vi "Lockin.Read Configuration.vi"(8 "error in (no error)":errorcluster, 11 "Instrument.Lockin":refnum<class "Instrument.Lockin.lvclass">) -> (0 "error out":errorcluster, 2 "Configuration":T1={"Channels: AO"={"Ch"=[], "Amp (V)"=[], "DC (V)"=[], "f (Hz)"=[], "Phase (°)"=[], "Function"=[], "Sweep?"=[]}, "Channels: REF"={"Ch"=[13], " f (Hz)"=[], "Phase (°)"=[], "TC (s)"=[0.0], "order"=[0]}, "REF Filter"={"60 Hz prefilter"=FALSE, "LP prefilter"=FALSE, "LP cutoff (Hz)"=0.0}, "Amplifers"={"offsets"=[], "Gain"=[], "Amplifiers"=enum."Manual"}, "DAQ"={"sampling"={"Fs"=0.0, "#s"=500}, "sample mode"=10178, "buffer size (S)"=0, "decimation"=0}, "Calibration"={"Cal Info"=[]}, "AI Configuration"=[], "AO Configuration"=[], "Aux Channel"="Dev2/ao0"} {"AO Configuration"."output terminal configuration" items=["Default"=-1, "RSE"=10083, "Differential"=10106, "Pseudodifferential"=12529]; "AI Configuration"."input terminal configuration" items=["default"=-1, "RSE"=10083, "NRSE"=10078, "Differential"=10106, "Pseudodifferential"=12529]; "AI Configuration"."AI.Coupling" items=["AC"=10045, "DC"=10050, "GND"=10066]; "DAQ"."sample mode" items=["Finite Samples"=10178, "Continuous Samples"=10123]; "Channels: AO"."f (Hz)" min=0.001 max=10000.0 format="%.3g"; "Channels: AO"."Phase (°)" format="%.3g"; "Channels: AO"."DC (V)" format="%.3p"; "Channels: AO"."Amp (V)" min=0.0 max=10.0 format="%.3p"; "Channels: REF"."order" min=1; "Channels: REF"."TC (s)" min=1e-05 format="%#_3p"; "Channels: REF"."Phase (°)" format="%.3g"; "Channels: REF"."f (Hz)" format="%.3g"}, 3 "Instrument.Lockin out":refnum<class "Instrument.Lockin.lvclass">)   [LabVIEW 2016, in "Instrument.Lockin.lvclass"]
uses:
  Instrument.Lockin.lvclass
  Typedefs/Lockin.Configuration--Cluster.ctl
  LockinDAQ/Typedefs/AO-cluster.ctl
  LockinDAQ/Typedefs/Function-enum.ctl
  LockinDAQ/Typedefs/REF-cluster.ctl
  LockinDAQ/Typedefs/AI Prefilter-cluster.ctl
  LockinDAQ/Typedefs/AmplifierType-enum.ctl
  LockinDAQ/Typedefs/Sampling.ctl
  LockinDAQ/Typedefs/Cal Info - Cluster.ctl
  LockinDAQ/Typedefs/AI.config-array.ctl
  LockinDAQ/Typedefs/AI.config-cluster.ctl
  LockinDAQ/Typedefs/AI.coupling-enum.ctl
  LockinDAQ/Typedefs/446xAI-enum.ctl
  LockinDAQ/Typedefs/DAQType-enum.ctl
  LockinDAQ/Typedefs/AO.config-array.ctl
  LockinDAQ/Typedefs/AO.config-cluster.ctl
  LockinDAQ/Typedefs/446xAO-enum.ctl
  Instrument.Lockin.lvclass/Instrument.Lockin.ctl
  LockinDAQ/LockinDAQ.lvclass
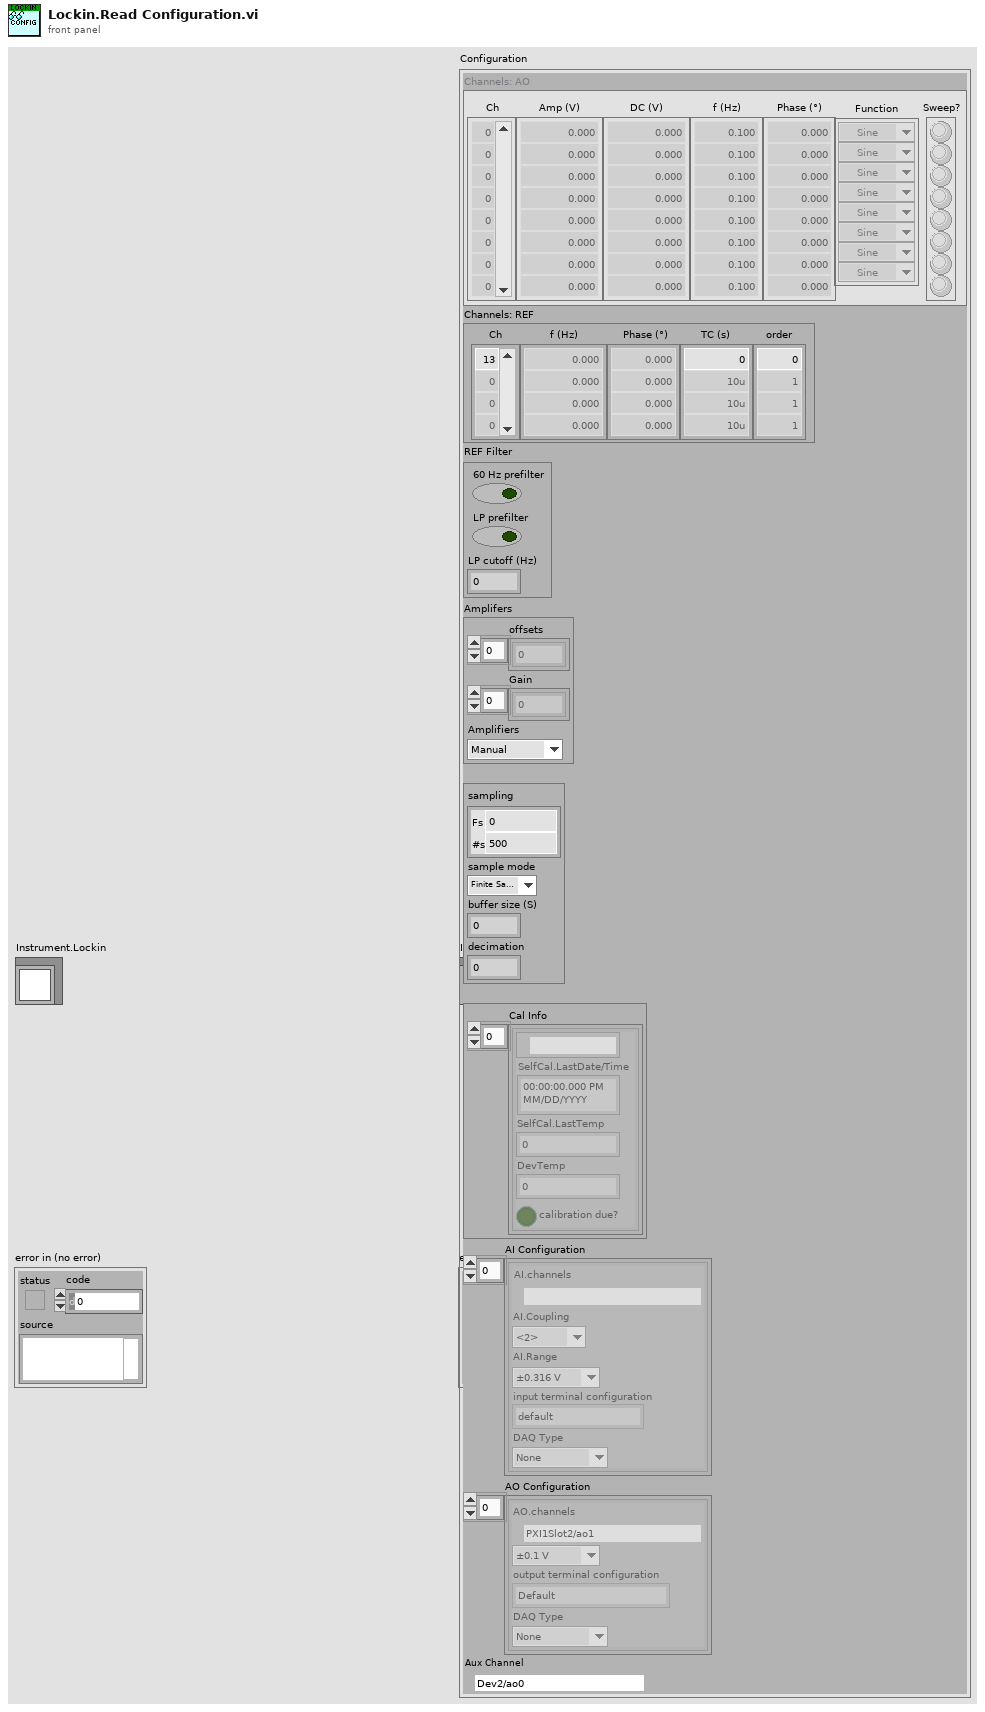
[diagram p1: front panel]
types:
  T1 = typedef "Instrument.Lockin.lvclass/Lockin.Configuration--Cluster.ctl" = cluster{"Channels: AO":T2, "Channels: REF":T4, "REF Filter":T5, "Amplifers":cluster{"offsets":dbl[], "Gain":dbl[], "Amplifiers":T6}, "DAQ":cluster{"sampling":T7, "sample mode":i32, "buffer size (S)":u32, "decimation":u32}, "Calibration":cluster{"Cal Info":T8[]}, "AI Configuration":T9, "AO Configuration":T14, "Aux Channel":tag}
  T2 = typedef "LockinDAQ.lvclass/AO-cluster.ctl" = cluster{"Ch":i32[], "Amp (V)":dbl[], "DC (V)":dbl[], "f (Hz)":dbl[], "Phase (°)":dbl[], "Function":T3[], "Sweep?":bool[]}
  T3 = typedef "LockinDAQ.lvclass/Function-enum.ctl" = enum16{"Sine", "Triangle", "Square", "Sawtooth"}
  T4 = typedef "LockinDAQ.lvclass/REF-cluster.ctl" = cluster{"Ch":i32[], " f (Hz)":dbl[], "Phase (°)":dbl[], "TC (s)":dbl[], "order":i32[]}
  T5 = typedef "LockinDAQ.lvclass/AI Prefilter-cluster.ctl" = cluster{"60 Hz prefilter":bool, "LP prefilter":bool, "LP cutoff (Hz)":dbl}
  T6 = typedef "LockinDAQ.lvclass/AmplifierType-enum.ctl" = enum16{"Manual", "Krohn Hite", "Femto"}
  T7 = typedef "LockinDAQ.lvclass/Sampling.ctl" = cluster{"Fs":dbl, "#s":i32}
  T8 = typedef "LockinDAQ.lvclass/Cal Info - Cluster.ctl" = cluster{"Active Device":tag, "SelfCal.LastDate/Time":timestamp, "SelfCal.LastTemp":dbl, "DevTemp":dbl, "calibration due?":bool}
  T9 = typedef "LockinDAQ.lvclass/AI.config-array.ctl" = T10[]
  T10 = typedef "LockinDAQ.lvclass/AI.config-cluster.ctl" = cluster{"AI.channels":tag, "AI.Coupling":T11, "AI.Range":T12, "input terminal configuration":i32, "DAQ Type":T13}
  T11 = typedef "LockinDAQ.lvclass/AI.coupling-enum.ctl" = u16
  T12 = typedef "LockinDAQ.lvclass/446xAI-enum.ctl" = enum16{"±0.316 V", "±1.00 V", "±3.16 V", "±10.0 V", "±31.6 V", "±42.4 V"}
  T13 = typedef "LockinDAQ.lvclass/DAQType-enum.ctl" = enum16{"None", "USB 4431", "PXI 446x"}
  T14 = typedef "LockinDAQ.lvclass/AO.config-array.ctl" = T15[]
  T15 = typedef "LockinDAQ.lvclass/AO.config-cluster.ctl" = cluster{"AO.channels":tag, "AO.Range":T16, "output terminal configuration":i32, "DAQ Type":T13}
  T16 = typedef "LockinDAQ.lvclass/446xAO-enum.ctl" = enum16{"±0.1 V", "±1.0 V", "±10.0 V"}
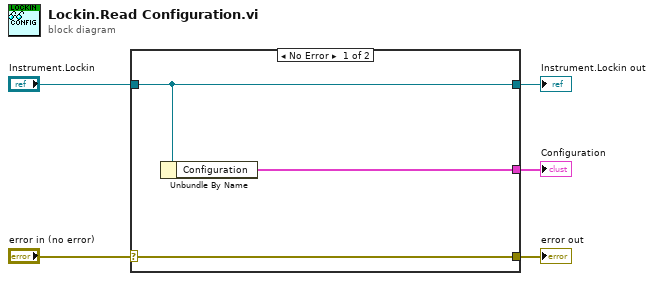
[diagram p0: block diagram]
diagram:
  n1 = case shown="No Error" "error in (no error)" {
    selector: "error in (no error)" -> [w8 w9]
    tunnel: [w8 w9] -> w4
    tunnel: [w7 w10] -> w2
    tunnel: "Instrument.Lockin" -> [w7 w10]
    tunnel: [w6 _] -> w1
    frame No Error {
      n2 = Unbundle By Name(w7) -> ("Configuration"=w6:T1)
    }
    frame Error {
    }
  }
  "error out" <- w4
  "Instrument.Lockin out" <- w2
  "Configuration" <- w1
